vi "Message to uService.vi"(0 "Guardian in":refnum<class "Guardian.lvclass">, 5 "uService ID":string, 7 "Message":string, 9 "Data":variant, 11 "error in (no error)":errorcluster, 12 "Locale?":bool) -> (4 "Guardian out":refnum<class "Guardian.lvclass">, 15 "error out":errorcluster)   [LabVIEW 2026, in "TALOS.lvlib" / "Guardian.lvlib" / "Guardian.lvclass"]
doc: "This VI sends a Message to the uService specified in uService ID. If the flag In locale? = True, it will try to locate it in locale and send a local message, or give an error; if the In locale? = False, it will search in the Distributed uService List and send it to all the Guardian s that are running an instance of that uService, comprised the local Guardian, if it is the case."
uses:
  Guardian.lvclass
  C:/LabVIEW Code/TALOS/talos/Ancestor/Ancestor/Ancestor.lvclass
  Ancestor/Ancestor/Ancestor.lvclass/Ancestor.ctl
  Father of all uServices/Father of all uServices/Event Handler Items.ctl
  Classes/uService List/uService List.lvclass/uService List.ctl
  Father of all uServices/Father of all uServices Messages/Event Handler Msg/Event Handler Msg.lvclass/Event Handler Msg.ctl
  Ancestor/Ancestor/Read ID.vi
  Ancestor/Ancestor/Read Distr uS Map ref.vi
  Classes/uService List/Get Queue.vi
  Support VIs/Generate Error.vi
  FGV/Error Memory/Get Error Description.vi
  Support VIs/Get PC name.vi
  Support VIs/Get Class Name.vi
  <vilib>/Utility/error.llb/Clear Errors.vi
  FGV/Error Memory/Error Memory Core.vi
  <vilib>/AdvancedString/Delimited String to 1D String Array.vi
  <vilib>/AdvancedString/Delimited String to 1D String Array (string).vi
  Support VIs/Circus Root Path.vi
  FGV/Error Memory/Error Crt Lvl checker.vi
  FGV/Error Memory/Error Memory Core.vi/40c8088d-b597-4017-91af-faa98e00292e.vi
  FGV/Error Memory/Error Memory Core.vi/d4a3ab98-063c-4e44-b43d-fbdcfe6c2be2.vi
  Support VIs/Global Constants.vi
  Support VIs/Global Memory.vi
  <vilib>/Utility/LVClass/Get LV Class Name.vi
  Support VIs/Is in Packed Library.vi
  Support VIs/TALOS Root path.vi
  Support VIs/Read CSV worksheet.vi
  <vilib>/Utility/error.llb/General Error Handler.vi
  builds/Actor Framework PPL/Actor Framework.lvlibp/1abvi3w/vi.lib/ActorFramework/Message Enqueuer/Enqueue.vi
  Support VIs/Error Log.vi
  Classes/Distributed uService Map/Distributed uService Map.lvclass
  builds/Actor Framework PPL/Actor Framework.lvlibp/1abvi3w/vi.lib/ActorFramework/Message Enqueuer/Message Enqueuer.lvclass
  Ancestor/Ancestor/Ancestor.lvclass
  <vilib>/Comparison/Equal/Equal Functor/Equal Functor.lvclass
  Father of all uServices/Father of all uServices Messages/Event Handler Msg/Event Handler Msg.lvclass
  Father of all uServices/Father of all uServices/Father of all uServices.lvclass
  Classes/uService List/uService List.lvclass
  TALOS.lvlib
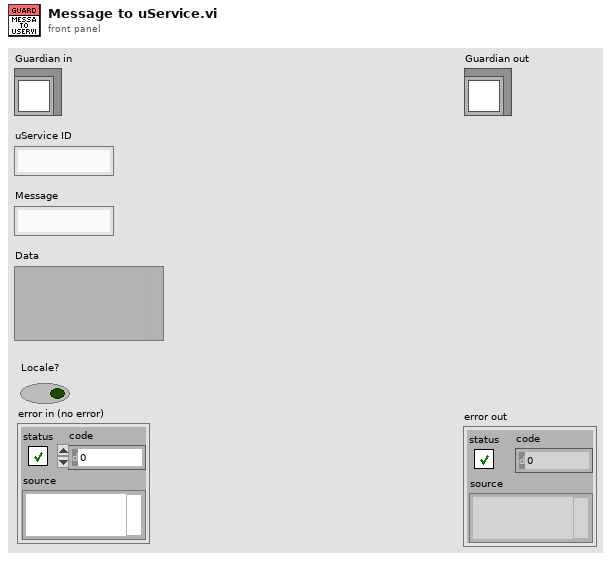
[diagram p1: front panel]
types:
  T1 = typedef "TALOS.lvlib/Father of all uServices.lvlib/Father of all uServices.lvclass/Event Handler Items.ctl" = enum16{"Button Pressed", "Message", "Ready to launch?", "Safe Mode", "Start RUN", "Stop RUN"}
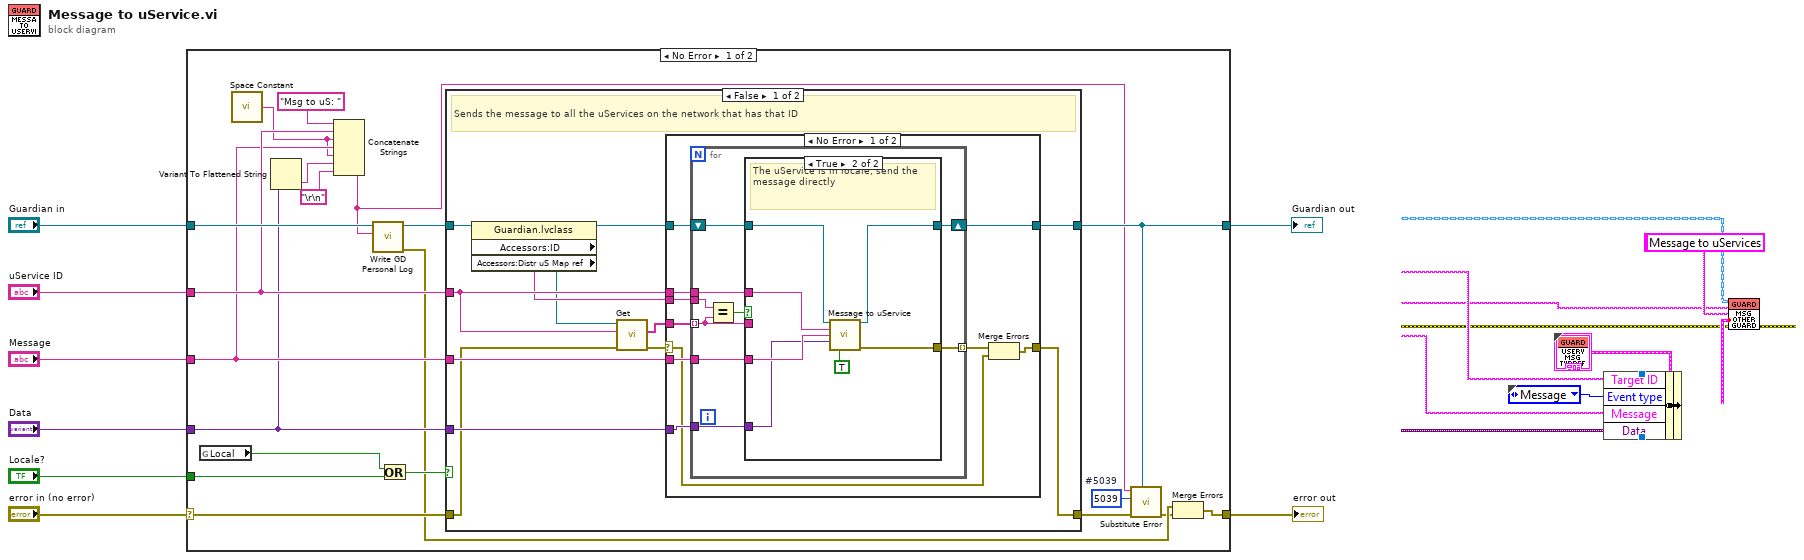
[diagram p0: block diagram]
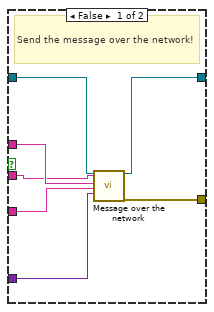
[diagram p2: hidden frame]
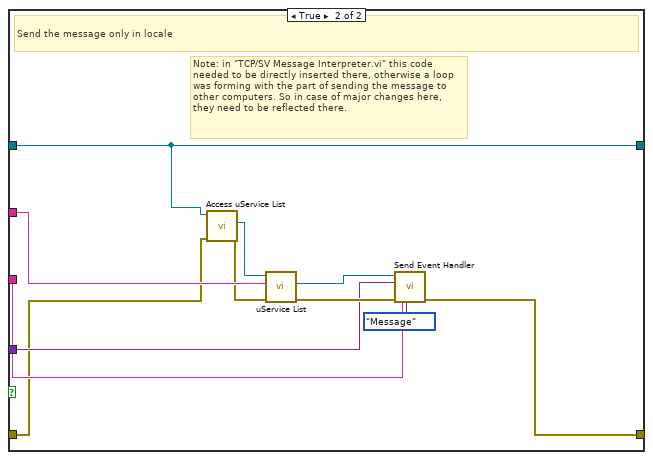
[diagram p4: hidden frame]
diagram:
  n1 = case shown="No Error" "error in (no error)" {
    selector: "error in (no error)" -> [w28 w88]
    tunnel: [w15 w88] -> w7
    tunnel: "uService ID" -> [w20 _]
    tunnel: "Data" -> [w18 _]
    tunnel: "Message" -> [w19 _]
    tunnel: "Locale?" -> [w26 _]
    tunnel: "Guardian in" -> [w23 w87]
    tunnel: [w11 w87] -> w1
    frame No Error {
      w9 = 5039  # #5039
      n2 = global read "Global Constants.vi" "Local"() -> (w27:bool)
      n3 = call <vilib>:"Space Constant.vi"() -> ("String"=w17:string)
      n4 = Variant To Flattened String(Variant=w18) -> (data string=w21:string)  [unwired: 1 out]
      n5 = Concatenate Strings("Msg to uS: " ("string"), w20, w17, w19, w17, w21, "\r\n") -> (w10:string)
      n6 = call "Write GD Personal Log.vi"("String"=w10, "Guardian in"=w23) -> ("error out"=w14:errorcluster, "Guardian out"=w24:refnum<class "Guardian.lvclass">)  [unwired: 8 in]
      n7 = Or(x=w27, y=w26) -> (x .or. y?=w25:bool)
      n8 = case shown="False" w25 {
        tunnel: w28 -> [w29 w77]
        tunnel: [w38 w76] -> w13
        tunnel: w20 -> [w36 w81]
        tunnel: w18 -> [w39 w84]
        tunnel: w19 -> [w40 w83]
        tunnel: w24 -> [w30 w80]
        tunnel: [w37 w80] -> w11
        frame False {
          # "Sends the message to all the uServices on the network that has that ID"
          n9 = property class="Guardian.lvclass"(reference=w30) -> (reference out=w33:refnum<class "Guardian.lvclass">, "Accessors:ID"=w32:string, "Accessors:Distr uS Map ref"=w31:refnum<data-value>)  [unwired: 1 in, 1 out]
          n10 = call "Get.vi"("error in (no error)"=w29, "uService ID"=w36, "Distr uS Map ref in"=w31) -> ("error out"=w35:errorcluster, "Guardians"=w34:string[])  [unwired: 5 in, 2 out]
          n11 = case shown="No Error" w35 {
            selector: w35 -> [w41 w74]
            tunnel: w34 -> [w50 _]
            tunnel: w32 -> [w49 _]
            tunnel: w36 -> [w48 _]
            tunnel: w40 -> [w47 _]
            tunnel: w39 -> [w46 _]
            tunnel: [w44 w74] -> w38
            tunnel: w33 -> [w43 w75]
            tunnel: [w42 w75] -> w37
            frame No Error {
              n12 = for {
                tunnel: w50 -> [w52] mode=indexing
                tunnel: w49 -> [w59]
                tunnel: w48 -> [w55]
                tunnel: w47 -> [w57]
                tunnel: w46 -> [w56]
                tunnel: [w54] -> w45 mode=indexing
                shift-right: [w51] -> w42
                shift-left: w43 -> [w53]
                n13 = Equal?(x=w59, y=w52) -> (x = y?=w58:bool)
                n14 = case shown="True" w58 {
                  tunnel: w57 -> [w62 w68]
                  tunnel: w56 -> [w61 w67]
                  tunnel: w55 -> [w63 w69]
                  tunnel: [w64 w73] -> w54
                  tunnel: w53 -> [w66 w70]
                  tunnel: w52 -> [w60 _]
                  tunnel: [w65 w71] -> w51
                  frame False {
                    # "Send the message over the network!"
                    n15 = call "Message over the network.vi"("Guardian in"=w66, "Destination GD ID"=w60, "Target ID (uService ID or \"Guardian\")"=w63, "Message"=w62, "Data"=w61) -> ("Guardian out"=w65:refnum<class "Guardian.lvclass">, "error out"=w64:errorcluster)  [unwired: 13 in]
                  }
                  frame True {
                    # "The uService is in locale, send the message directly"
                    n16 = call "Message to uService.vi"("Guardian in"=w70, "uService ID"=w69, "Message"=w68, "Data"=w67, "Locale?"=TRUE) -> ("Guardian out"=w71:refnum<class "Guardian.lvclass">, "error out"=w73:errorcluster)  [unwired: 9 in]
                  }
                }
              }
              n17 = Merge Errors(w45, w41) -> (w44:errorcluster)
            }
            frame Error {
            }
          }
        }
        frame True {
          # "Note: in \"TCP/SV Message Interpreter.vi\" this code needed to be directly inserted there, otherwise a loop was forming with the part of sending the message to other computers. So in case of major changes here, they need to be reflected there."
          # "Send the message only in locale"
          n18 = call-dynamic "Access uService List.vi"("error in (no error)"=w77, "Ancestor in"=w80) -> ("error out"=w78:errorcluster, "uService List out"=w79:refnum<class "uService List.lvclass">)  [unwired: 7 in, 1 out]
          n19 = call-poly "uService List.vi"("error in (no error)"=w78, "ID"=w81, "uService List in"=w79) -> ("error out"=w86:errorcluster, "uService Queue"=w82:refnum<class "Message Enqueuer.lvclass">)  [unwired: 6 in, 1 out]
          n20 = call "Send Event Handler.vi"("Event type"=Event_Handler_Items."Message", "error in (no error)"=w86, "Item Name"=w83, "Data"=w84, "Message Enqueuer"=w82) -> ("error out"=w76:errorcluster)  [unwired: 5 in, 1 out]
        }
      }
      n21 = call "Substitute Error.vi"("LabVIEW Object"=w11, "error in (no error)"=w13, "Error Code"=w9, "Optional String"=w10) -> ("error out"=w12:errorcluster)  [unwired: 7 in]
      n22 = Merge Errors(w14, w12) -> (w15:errorcluster)
    }
    frame Error {
    }
  }
  "error out" <- w7
  "Guardian out" <- w1
